vi "WriteConfigFile.vi"(8 "error in (no error)":errorcluster, 11 "MFActor in":refnum<class "MFActor.lvclass">) -> (0 "error out":errorcluster, 3 "MFActor out":refnum<class "MFActor.lvclass">)   [LabVIEW 2024, in "MFActor.lvlib" / "MFActor.lvclass"]
uses:
  MFActor.lvclass
  MFActor.lvclass/MFActor.ctl
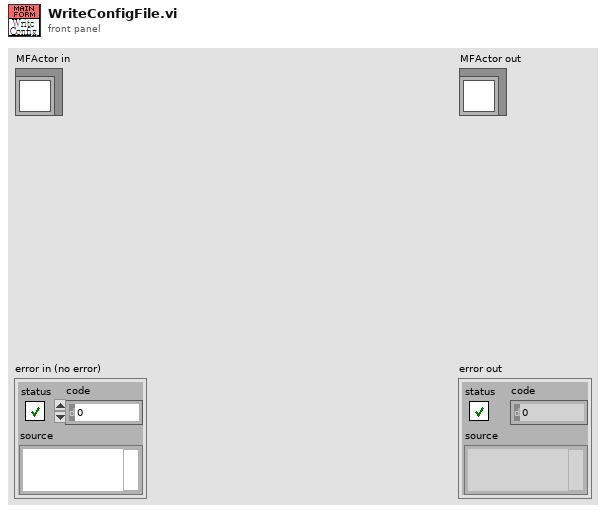
[diagram p1: front panel]
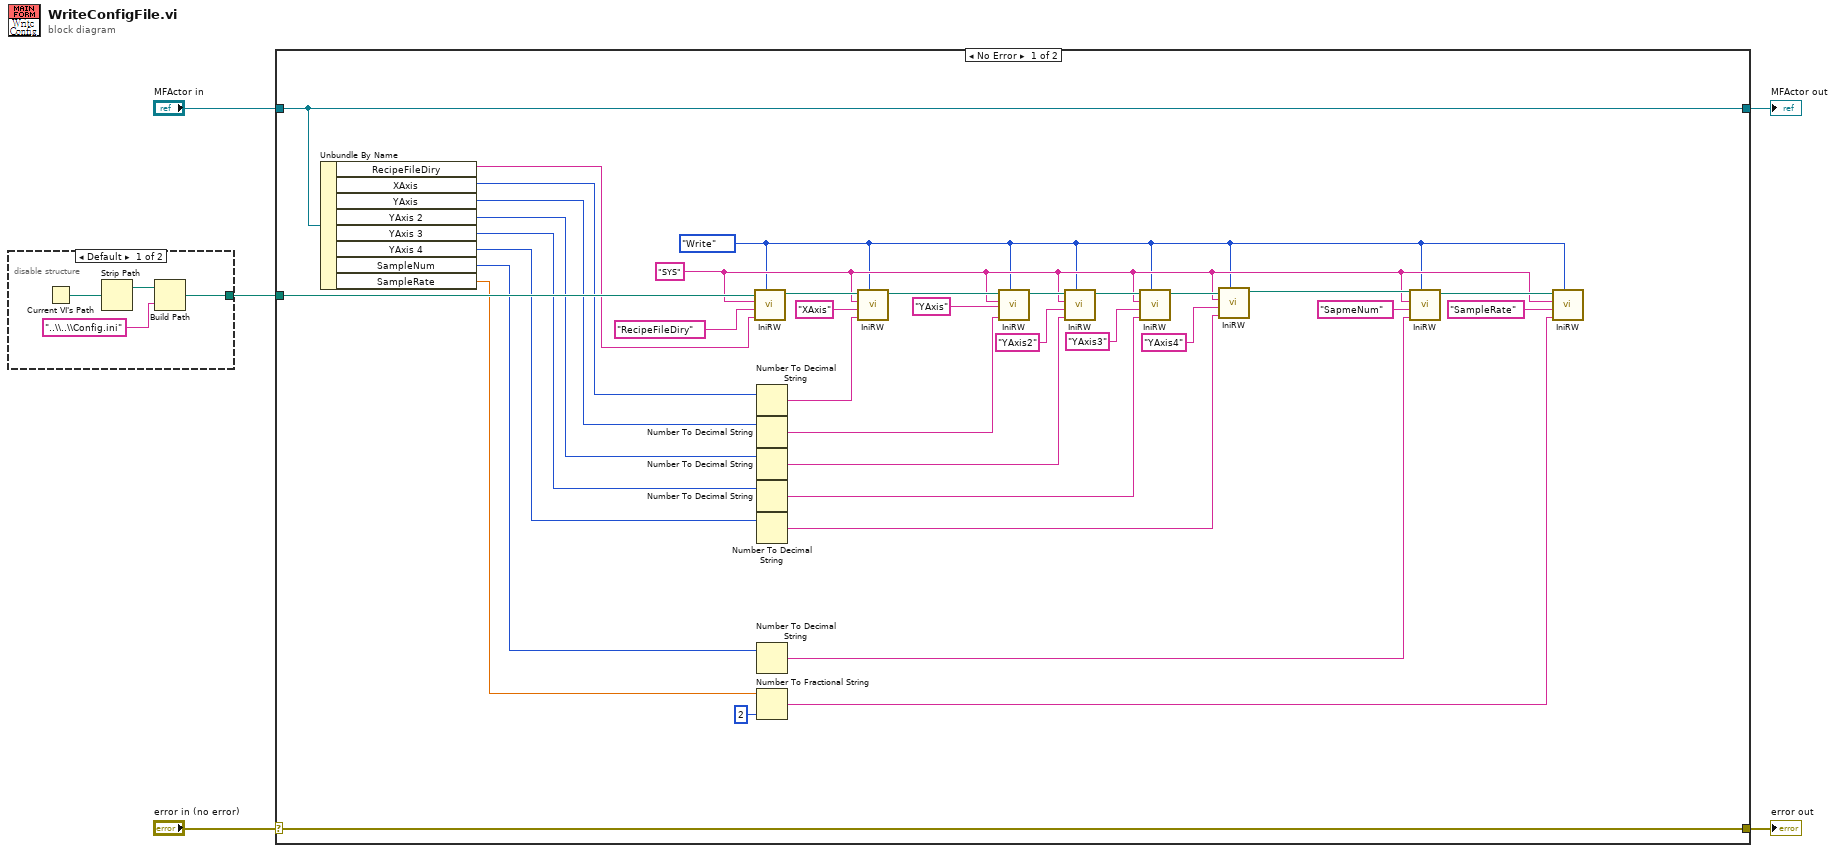
[diagram p0: block diagram]
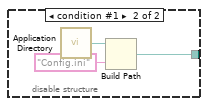
[diagram p2: hidden frame]
diagram:
  n1 = disable-structure shown="Default" {
    disable-tunnel: [w6 w10] -> w1
    frame condition #0 (active) {
      n2 = Current VI's Path() -> (path=w9:path)
      n3 = Strip Path(path=w9) -> (stripped path=w8:path)  [unwired: 1 out]
      n4 = Build Path(base path=w8, name or relative path="..\\..\\Config.ini") -> (appended path=w6:path)
    }
    frame condition #1 {
      n5 = call <vilib>:"Application Directory.vi"() -> ("Application Directory"=w12:path)
      n6 = Build Path(base path=w12, name or relative path="Config.ini") -> (appended path=w10:path)
    }
  }
  n7 = case shown="No Error" "error in (no error)" {
    selector: "error in (no error)" -> [w48 w50]
    tunnel: [w48 w50] -> w4
    tunnel: [w45 w49] -> w2
    tunnel: "MFActor in" -> [w45 w49]
    tunnel: w1 -> [w46 _]
    frame No Error {
      w19 = enum16{"None", "Read", "Write"}."Write" ("Operation")
      w20 = "SYS"
      n8 = Unbundle By Name(w45) -> ("RecipeFileDiry"=w44:string, "XAxis"=w43:u16, "YAxis"=w42:u16, "YAxis 2"=w15:u16, "YAxis 3"=w14:u16, "YAxis 4"=w13:u16, "SampleNum"=w41:u32, "SampleRate"=w40:dbl)
      n9 = call "IniRW.vi"("Operation"=w19, "InputValue"=w44, "Key"="RecipeFileDiry", "Section"=w20, "IniFilePath"=w46) -> ("IniFilePath out"=w38:path)  [unwired: 4 in, 2 out]
      n10 = Number To Decimal String(number=w43) -> (decimal integer string=w31:string)  [unwired: 1 in]
      n11 = Number To Decimal String(number=w42) -> (decimal integer string=w30:string)  [unwired: 1 in]
      n12 = Number To Decimal String(number=w15) -> (decimal integer string=w23:string)  [unwired: 1 in]
      n13 = Number To Decimal String(number=w14) -> (decimal integer string=w22:string)  [unwired: 1 in]
      n14 = Number To Decimal String(number=w13) -> (decimal integer string=w21:string)  [unwired: 1 in]
      n15 = Number To Decimal String(number=w41) -> (decimal integer string=w29:string)  [unwired: 1 in]
      n16 = Number To Fractional String(number=w40, precision (6)=i16 2) -> (F-format string=w28:string)  [unwired: 2 in]
      n17 = call "IniRW.vi"("Operation"=w19, "InputValue"=w31, "Key"="XAxis", "Section"=w20, "IniFilePath"=w38) -> ("IniFilePath out"=w37:path)  [unwired: 4 in, 2 out]
      n18 = call "IniRW.vi"("Operation"=w19, "InputValue"=w30, "Key"="YAxis", "Section"=w20, "IniFilePath"=w37) -> ("IniFilePath out"=w27:path)  [unwired: 4 in, 2 out]
      n19 = call "IniRW.vi"("Operation"=w19, "InputValue"=w23, "Key"="YAxis2", "Section"=w20, "IniFilePath"=w27) -> ("IniFilePath out"=w26:path)  [unwired: 4 in, 2 out]
      n20 = call "IniRW.vi"("Operation"=w19, "InputValue"=w22, "Key"="YAxis3", "Section"=w20, "IniFilePath"=w26) -> ("IniFilePath out"=w25:path)  [unwired: 4 in, 2 out]
      n21 = call "IniRW.vi"("Operation"=w19, "InputValue"=w21, "Key"="YAxis4", "Section"=w20, "IniFilePath"=w25) -> ("IniFilePath out"=w24:path)  [unwired: 4 in, 2 out]
      n22 = call "IniRW.vi"("Operation"=w19, "InputValue"=w29, "Key"="SapmeNum", "Section"=w20, "IniFilePath"=w24) -> ("IniFilePath out"=w33:path)  [unwired: 4 in, 2 out]
      n23 = call "IniRW.vi"("Operation"=w19, "InputValue"=w28, "Key"="SampleRate", "Section"=w20, "IniFilePath"=w33) -> ()  [unwired: 4 in, 3 out]
    }
    frame Error {
    }
  }
  "error out" <- w4
  "MFActor out" <- w2
